vi "Day 3-2.vi"() -> ()   [LabVIEW 2019, in "Day 3.lvlib"]
uses:
  Day 3.lvlib
panel:
  out "Result":u32
  out "CO2":u32
  out "Oxigen":u32
  in  "String":string="010110011101\n101100111000\n100100000011\n111000010001\n001100010011\n010000111100\n001000100011\n001000100111\n010001111110\n111101001011\n011000101011\n111100111001\n100101111011\n101100110110\n101010111001\n001111000110\n001001101000\n101011001010\n011101111010\n011101001010\n011001000001\n100001010000\n111011001101\n000111110111\n010011001111\n000111011001\n111000010100\n101001100100\n110010001101\n111110101000\n011001100010\n110010110101\n010000001101\n100000000100\n110111011110\n110001100110\n001011110111\n110000011110\n110110101010\n101001100110\n010000001010\n100010100100\n101000111101\n111000001011\n000000100100\n100111010110\n01..."
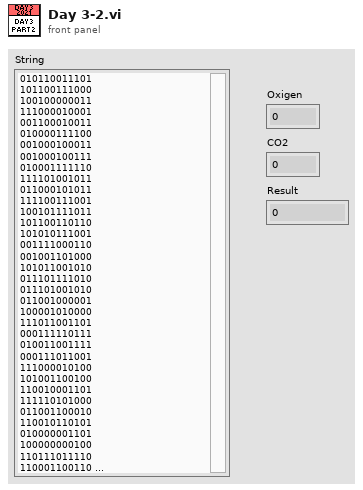
[diagram p1: front panel]
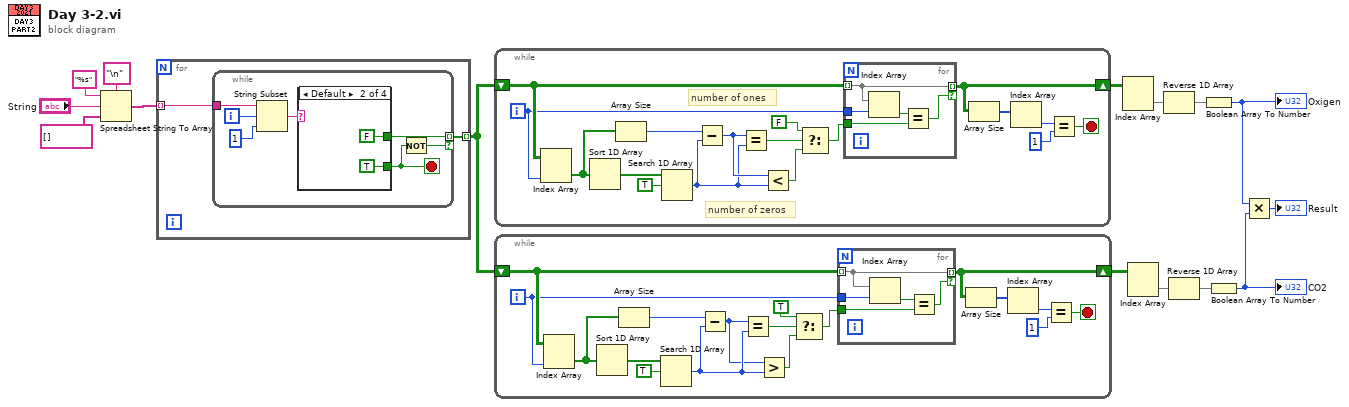
[diagram p0: block diagram]
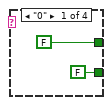
[diagram p2: hidden frame]
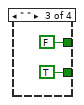
[diagram p3: hidden frame]
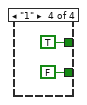
[diagram p4: hidden frame]
diagram:
  n1 = Spreadsheet String To Array(delimiter (Tab)="\n", format string="%s", spreadsheet string="String", array type (2D Dbl)=string[] []) -> (array=w1:string[])
  n2 = for {
    tunnel: w1 -> [w17] mode=indexing
    tunnel: [w16] -> w10 mode=indexing
    n3 = while {
      tunnel: w17 -> [w24]
      tunnel: [w20] -> w16 mode=indexing if=w19
      i -> [w23]
      stop <- w18 stop-if-true
      n4 = String Subset(string=w24, offset (0)=w23, length (rest)=1 ("length (rest)")) -> (substring=w21:string)
      n5 = case shown="Default" w21 {
        tunnel: [FALSE FALSE FALSE TRUE] -> w20
        tunnel: [FALSE TRUE TRUE FALSE] -> w18
        frame "0" {
        }
        frame Default {
        }
        frame " " {
        }
        frame "1" {
        }
      }
      n6 = Not(x=w18) -> (.not. x?=w19:bool)
    }
  }
  n7 = while {
    shift-right: [w34] -> w7
    shift-left: w10 -> [w49]
    i -> [w33]
    stop <- w45 stop-if-true
    # "number of ones"
    # "number of zeros"
    n8 = Index Array(array=w49, index (col)=w33) -> (element=w44:bool[])  [unwired: 1 in]
    n9 = Sort 1D Array(array=w44) -> (sorted array=w42:bool[])
    n10 = Array Size(array=w44) -> (size(s)=w38:i32)
    n11 = Search 1D Array(1D array=w42, element=TRUE) -> (index of element=w35:i32)  [unwired: 1 in]
    n12 = Subtract(x=w38, y=w35) -> (x-y=w36:i32)
    n13 = Equal?(x=w36, y=w35) -> (x = y?=w41:bool)
    n14 = Less?(x=w36, y=w35) -> (x < y?=w37:bool)
    n15 = Select(t=FALSE, s=w41, f=w37) -> (s? t:f=w40:bool)
    n16 = for {
      tunnel: w49 -> [w54] mode=indexing
      tunnel: [w54] -> w34 mode=indexing if=w51
      tunnel: w40 -> [w52]
      tunnel: w33 -> [w50]
      n17 = Index Array(array=w54, index=w50) -> (element=w53:bool)
      n18 = Equal?(x=w53, y=w52) -> (x = y?=w51:bool)
    }
    n19 = Array Size(array=w34) -> (size(s)=w48:i32[])
    n20 = Index Array(array=w48) -> (element=w47:i32)  [unwired: 1 in]
    n21 = Equal?(x=w47, y=1) -> (x = y?=w45:bool)
  }
  n22 = while {
    shift-right: [w60] -> w6
    shift-left: w10 -> [w71]
    i -> [w55]
    stop <- w67 stop-if-true
    n23 = Index Array(array=w71, index (col)=w55) -> (element=w66:bool[])  [unwired: 1 in]
    n24 = Sort 1D Array(array=w66) -> (sorted array=w64:bool[])
    n25 = Array Size(array=w66) -> (size(s)=w59:i32)
    n26 = Search 1D Array(1D array=w64, element=TRUE) -> (index of element=w58:i32)  [unwired: 1 in]
    n27 = Subtract(x=w59, y=w58) -> (x-y=w57:i32)
    n28 = Equal?(x=w57, y=w58) -> (x = y?=w62:bool)
    n29 = Greater?(x=w57, y=w58) -> (0:w56:bool)
    n30 = Select(t=TRUE, s=w62, f=w56) -> (s? t:f=w61:bool)
    n31 = for {
      tunnel: w71 -> [w76] mode=indexing
      tunnel: [w76] -> w60 mode=indexing if=w73
      tunnel: w61 -> [w74]
      tunnel: w55 -> [w72]
      n32 = Index Array(array=w76, index=w72) -> (element=w75:bool)
      n33 = Equal?(x=w75, y=w74) -> (x = y?=w73:bool)
    }
    n34 = Array Size(array=w60) -> (size(s)=w70:i32[])
    n35 = Index Array(array=w70) -> (element=w69:i32)  [unwired: 1 in]
    n36 = Equal?(x=w69, y=1) -> (x = y?=w67:bool)
  }
  n37 = Index Array(array=w7) -> (element=w11:bool[])  [unwired: 2 in]
  n38 = Index Array(array=w6) -> (element=w9:bool[])  [unwired: 2 in]
  n39 = Reverse 1D Array(array=w11) -> (reversed array=w12:bool[])
  n40 = Reverse 1D Array(array=w9) -> (reversed array=w8:bool[])
  n41 = Boolean Array To Number(Boolean array=w12) -> (number=w15:u32)
  "Oxigen" <- w15
  n42 = Boolean Array To Number(Boolean array=w8) -> (number=w14:u32)
  "CO2" <- w14
  n43 = Multiply(x=w15, y=w14) -> (x*y=→"Result":u32)
